vi "CRC-MODBUS.vi"(1 "数据":string) -> (0 "数据+CRC":string)   [LabVIEW 2019]
panel:
  out "hex integer string":string
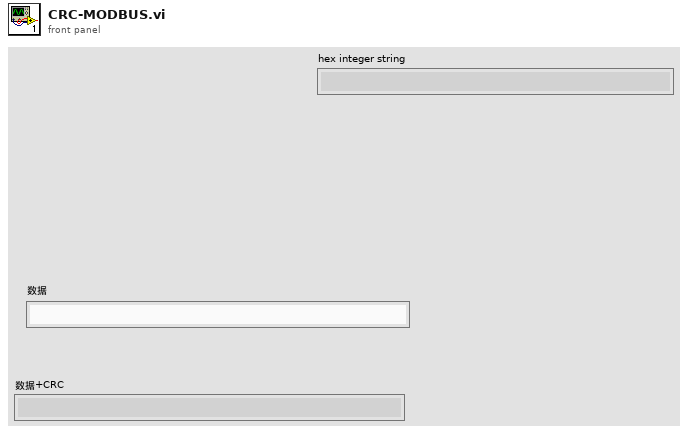
[diagram p1: front panel]
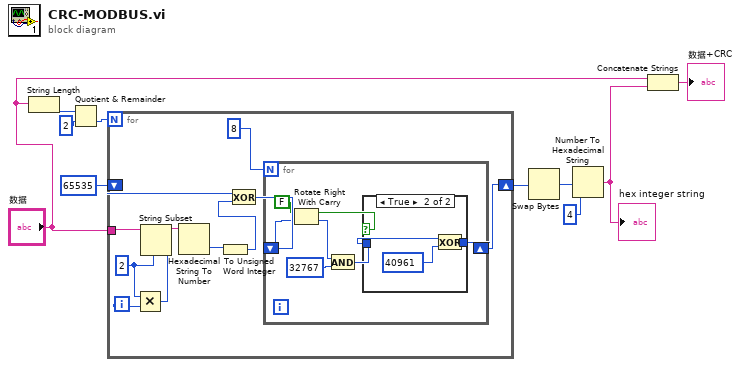
[diagram p0: block diagram]
diagram:
  n1 = String Length(string="数据") -> (length=w7:i32)
  n2 = Quotient & Remainder(x=w7, y=2) -> (floor(x/y)=w5:i32)  [unwired: 1 out]
  n3 = for {
    N: w5 -> [_]
    shift-right: [w14] -> w8
    shift-left: 65535 -> [w21]
    tunnel: "数据" -> [w20]
    i -> [w19]
    w12 = 2
    n4 = Multiply(x=w12, y=w19) -> (x*y=w11:i32)
    n5 = String Subset(string=w20, offset (0)=w11, length (rest)=w12) -> (substring=w17:string)
    n6 = Hexadecimal String To Number(string=w17) -> (number=w16:u32)  [unwired: 2 in, 1 out]
    n7 = To Unsigned Word Integer(number=w16) -> (unsigned 16bit integer=w15:u16)
    n8 = Exclusive Or(1:w15, 2:w21) -> (0:w18:i32)
    n9 = for {
      N: 8 -> [_]
      shift-right: [w22] -> w14
      shift-left: w18 -> [w24]
      n10 = Rotate Right With Carry(2:w24, 3:FALSE) -> (0:w25:i32, 1:w26:bool)
      n11 = And(x=w25, y=32767) -> (x .and. y?=w27:i32)
      n12 = case shown="True" w26 {
        tunnel: w27 -> [w29 w31]
        tunnel: [w29 w30] -> w22
        frame False {
        }
        frame True {
          n13 = Exclusive Or(1:40961, 2:w31) -> (0:w30:i32)
        }
      }
    }
  }
  n14 = Swap Bytes(anything=w8) -> (byte swapped=w6:i32)
  n15 = Number To Hexadecimal String(1:i16 4 ("width (-)"), 2:w6) -> (0:w4:string)
  "hex integer string" <- w4
  n16 = Concatenate Strings("数据", w4) -> (→"数据+CRC":string)
